vi "Configure QuickDrop UI.vi"(6 "Type":T2=enum."Double Float", 7 "FP UI References":T1, 8 "error in (no error)":errorcluster, 10 "Operation":string) -> (0 "error out":errorcluster)   [LabVIEW 2016]
doc: "Dynamically shows or hides the relevant controls on the front panel of the Quick Drop UI, and renames some of the captions for controls to make it perform correctly."
uses:
  <vilib>/Utility/Data Type/Type Definitions/Data Type.ctl
  FP UI References.ctl
  Comparison Ctrl Refs.ctl
  Comparison Captions.ctl
  Comparison Visibility.ctl
  <vilib>/Utility/Data Type/NI_Data Type.lvlib
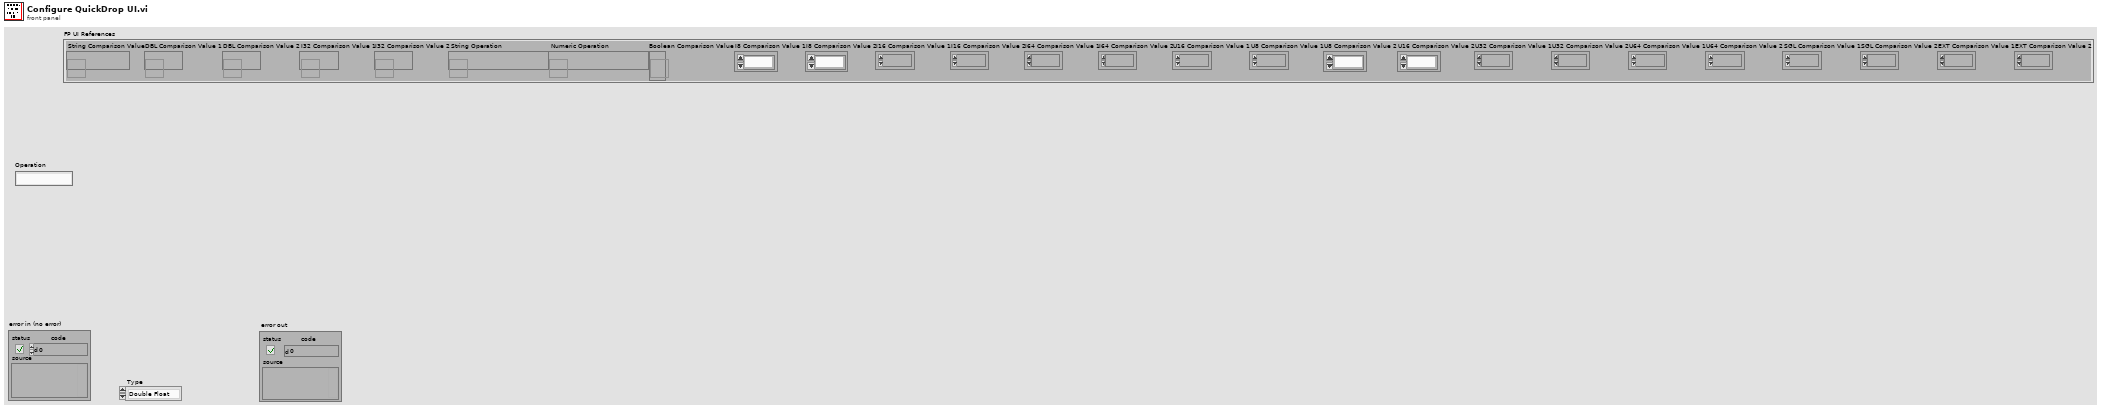
[diagram p1: front panel]
types:
  T1 = typedef "FP UI References.ctl" = cluster{"String Comparison Value":refnum<vi>, "DBL Comparison Value 1":refnum<vi>, "DBL Comparison Value 2":refnum<vi>, "I32 Comparison Value 1":refnum<vi>, "I32 Comparison Value 2":refnum<vi>, "String Operation":refnum<vi>, "Numeric Operation":refnum<vi>, "Boolean Comparison Value":refnum<vi>, "I8 Comparison Value 1":refnum<vi>, "I8 Comparison Value 2":refnum<vi>, "I16 Comparison Value 1":refnum<vi>, "I16 Comparison Value 2":refnum<vi>, "I64 Comparison Value 1":refnum<vi>, "I64 Comparison Value 2":refnum<vi>, "U16 Comparison Value 1":refnum<vi>, "U8 Comparison Value 1":refnum<vi>, "U8 Comparison Value 2":refnum<vi>, "U16 Comparison Value 2":refnum<vi>, "U32 Comparison Value 1":refnum<vi>, "U32 Comparison Value 2":refnum<vi>, "U64 Comparison Value 1":refnum<vi>, "U64 Comparison Value 2":refnum<vi>, "SGL Comparison Value 1":refnum<vi>, "SGL Comparison Value 2":refnum<vi>, "EXT Comparison Value 1":refnum<vi>, "EXT Comparison Value 2":refnum<vi>}
  T2 = typedef "NI_Data Type.lvlib/Data Type.ctl" = enum8{"Invalid Type", "Void", "I8", "I16", "I32", "I64", "U8", "U16", "U32", "U64", "Single Float", "Double Float", "Extended Float", "Single Complex", "Double Complex", "Extended Complex", "Enum U8", "Enum U16", "Enum U32", "Enum U64", "Single Float With Unit", "Double Float With Unit", "Extended Float With Unit", "Single Complex with Unit", "Double Complex with Unit", "Extended Complex with Unit", "Boolean", "String", "Path", "Picture", "Tag", "Array", "Cluster", "Variant", "LV Variant", "Waveform", "Timestamp", "Digital Waveform", "Digital Data", "ExpressData", "Refnum", "External Data", "VI", "Poly VI", "LabVIEW Class Instance", "Fixed Point"}
  T3 = typedef "Comparison Visibility.ctl" = cluster{"Comparison 2 Visible":bool, "Comparison 1 Visible":bool}
  T4 = typedef "Comparison Captions.ctl" = cluster{"Comparison 1 Caption":string, "Comparison 2 Caption":string}
  T5 = typedef "Comparison Ctrl Refs.ctl" = cluster{"Comparison Value 1 Control":refnum<vi>, "Comparison Value 2 Control":refnum<vi>}
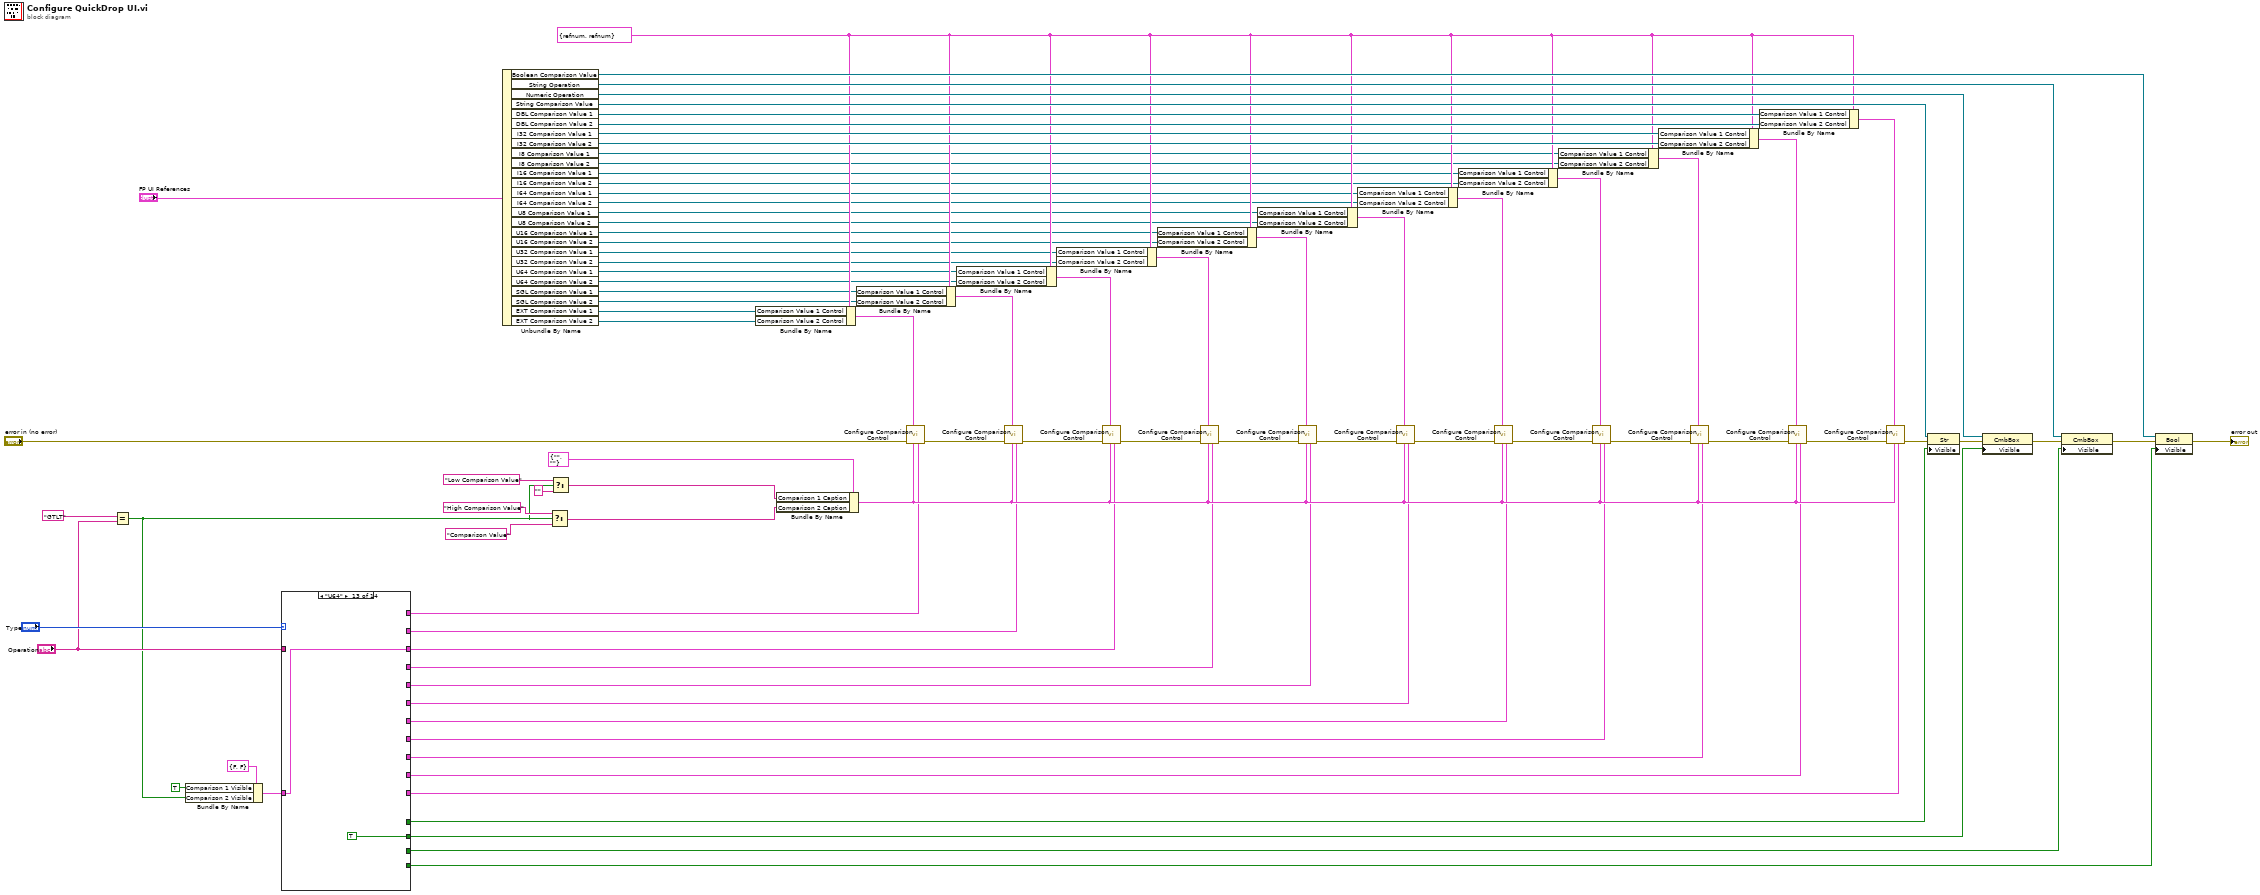
[diagram p0: block diagram]
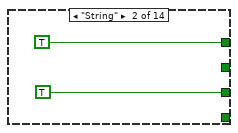
[diagram p3: hidden frame]
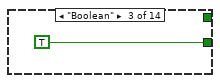
[diagram p4: hidden frame]
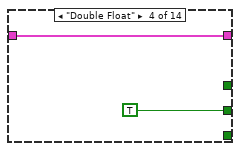
[diagram p5: hidden frame]
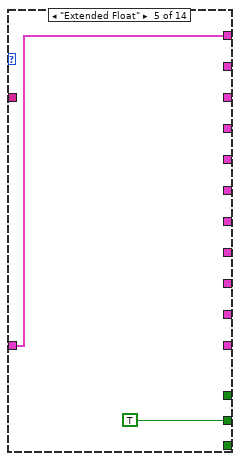
[diagram p6: hidden frame]
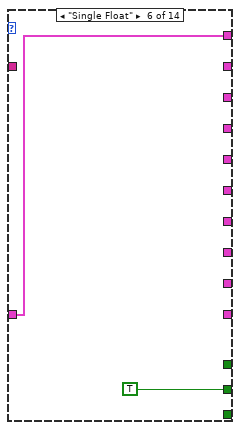
[diagram p7: hidden frame]
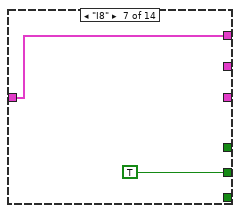
[diagram p8: hidden frame]
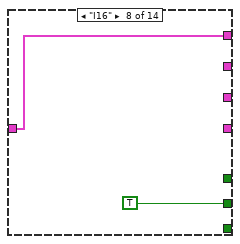
[diagram p9: hidden frame]
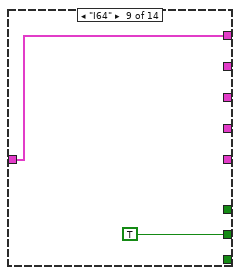
[diagram p10: hidden frame]
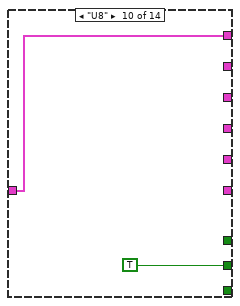
[diagram p11: hidden frame]
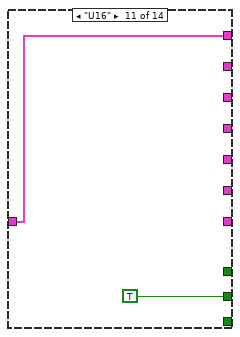
[diagram p12: hidden frame]
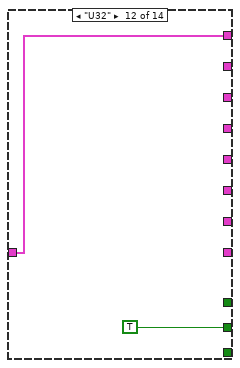
[diagram p13: hidden frame]
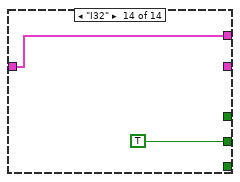
[diagram p14: hidden frame]
diagram:
  w55 = T5 {"Comparison Value 1 Control"=refnum, "Comparison Value 2 Control"=refnum} ("Control Refs")
  n1 = Equal?(x="GTLT", y="Operation") -> (x = y?=w2:bool)
  n2 = Bundle By Name(cluster=T3 {"Comparison 2 Visible"=FALSE, "Comparison 1 Visible"=FALSE} ("Control Visibility"), "Comparison 1 Visible"=TRUE, "Comparison 2 Visible"=w2) -> (w1:T3)
  n3 = case shown="\"U64\"" "Type" {
    tunnel: [_ TRUE _ _ _ _ _ _ _ _ _ _ _ _] -> w79
    tunnel: [_ TRUE _ _ _ _ _ _ _ _ _ _ _ _] -> w75
    tunnel: [_ _ _ TRUE TRUE TRUE TRUE TRUE TRUE TRUE TRUE TRUE TRUE TRUE] -> w74
    tunnel: "Operation" -> [_ _ _ _ _ _ _ _ _ _ _ _ _ _]
    tunnel: [_ _ TRUE _ _ _ _ _ _ _ _ _ _ _] -> w66
    tunnel: [_ _ _ _ w91 _ _ _ _ _ _ _ _ _] -> w15
    tunnel: [_ _ _ _ _ w93 _ _ _ _ _ _ _ _] -> w14
    tunnel: [_ _ _ _ _ _ _ _ _ _ _ _ w107 _] -> w13
    tunnel: [_ _ _ _ _ _ _ _ _ _ _ w105 _ _] -> w12
    tunnel: [_ _ _ _ _ _ _ _ _ _ w103 _ _ _] -> w11
    tunnel: [_ _ _ _ _ _ _ _ _ w101 _ _ _ _] -> w10
    tunnel: [_ _ _ _ _ _ _ _ w99 _ _ _ _ _] -> w9
    tunnel: [_ _ _ _ _ _ _ w97 _ _ _ _ _ _] -> w8
    tunnel: [_ _ _ _ _ _ w95 _ _ _ _ _ _ _] -> w7
    tunnel: [_ _ _ _ _ _ _ _ _ _ _ _ _ w109] -> w6
    tunnel: [_ _ _ w89 _ _ _ _ _ _ _ _ _ _] -> w5
    tunnel: w1 -> [_ _ _ w89 w91 w93 w95 w97 w99 w101 w103 w105 w107 w109]
    frame "Invalid Type", Default {
    }
    frame "String" {
    }
    frame "Boolean" {
    }
    frame "Double Float" {
    }
    frame "Extended Float" {
    }
    frame "Single Float" {
    }
    frame "I8" {
    }
    frame "I16" {
    }
    frame "I64" {
    }
    frame "U8" {
    }
    frame "U16" {
    }
    frame "U32" {
    }
    frame "U64" {
    }
    frame "I32" {
    }
  }
  n4 = Unbundle By Name("FP UI References") -> ("Boolean Comparison Value"=w67:refnum<vi>, "String Operation"=w76:refnum<vi>, "Numeric Operation"=w69:refnum<vi>, "String Comparison Value"=w83:refnum<vi>, "DBL Comparison Value 1"=w57:refnum<vi>, "DBL Comparison Value 2"=w56:refnum<vi>, "I32 Comparison Value 1"=w63:refnum<vi>, "I32 Comparison Value 2"=w62:refnum<vi>, "I8 Comparison Value 1"=w54:refnum<vi>, "I8 Comparison Value 2"=w53:refnum<vi>, "I16 Comparison Value 1"=w52:refnum<vi>, "I16 Comparison Value 2"=w51:refnum<vi>, "I64 Comparison Value 1"=w50:refnum<vi>, "I64 Comparison Value 2"=w49:refnum<vi>, "U8 Comparison Value 1"=w48:refnum<vi>, "U8 Comparison Value 2"=w47:refnum<vi>, "U16 Comparison Value 1"=w46:refnum<vi>, "U16 Comparison Value 2"=w45:refnum<vi>, "U32 Comparison Value 1"=w44:refnum<vi>, "U32 Comparison Value 2"=w43:refnum<vi>, "U64 Comparison Value 1"=w42:refnum<vi>, "U64 Comparison Value 2"=w41:refnum<vi>, "SGL Comparison Value 1"=w40:refnum<vi>, "SGL Comparison Value 2"=w39:refnum<vi>, "EXT Comparison Value 1"=w38:refnum<vi>, "EXT Comparison Value 2"=w37:refnum<vi>)
  n5 = Select(t="High Comparison Value", s=w2, f="Comparison Value") -> (s? t:f=w58:string)
  n6 = Select(t="Low Comparison Value", s=w2, f="") -> (s? t:f=w59:string)
  n7 = Bundle By Name(cluster=w55, "Comparison Value 1 Control"=w38, "Comparison Value 2 Control"=w37) -> (w17:T5)
  n8 = Bundle By Name(cluster=T4 {"Comparison 1 Caption"="", "Comparison 2 Caption"=""} ("Control Captions"), "Comparison 1 Caption"=w59, "Comparison 2 Caption"=w58) -> (w16:T4)
  n9 = Bundle By Name(cluster=w55, "Comparison Value 1 Control"=w40, "Comparison Value 2 Control"=w39) -> (w19:T5)
  n10 = call "Configure Comparison Control.vi"("Control Visibility"=w15, "Control Captions"=w16, "Control Refs"=w17, "error in (no error)"="error in (no error)") -> ("error out"=w18:errorcluster)  [unwired: 7 in]
  n11 = Bundle By Name(cluster=w55, "Comparison Value 1 Control"=w42, "Comparison Value 2 Control"=w41) -> (w20:T5)
  n12 = call "Configure Comparison Control.vi"("Control Visibility"=w14, "Control Captions"=w16, "Control Refs"=w19, "error in (no error)"=w18) -> ("error out"=w35:errorcluster)  [unwired: 7 in]
  n13 = Bundle By Name(cluster=w55, "Comparison Value 1 Control"=w44, "Comparison Value 2 Control"=w43) -> (w21:T5)
  n14 = call "Configure Comparison Control.vi"("Control Visibility"=w13, "Control Captions"=w16, "Control Refs"=w20, "error in (no error)"=w35) -> ("error out"=w28:errorcluster)  [unwired: 7 in]
  n15 = Bundle By Name(cluster=w55, "Comparison Value 1 Control"=w46, "Comparison Value 2 Control"=w45) -> (w22:T5)
  n16 = call "Configure Comparison Control.vi"("Control Visibility"=w12, "Control Captions"=w16, "Control Refs"=w21, "error in (no error)"=w28) -> ("error out"=w30:errorcluster)  [unwired: 7 in]
  n17 = Bundle By Name(cluster=w55, "Comparison Value 1 Control"=w48, "Comparison Value 2 Control"=w47) -> (w23:T5)
  n18 = call "Configure Comparison Control.vi"("Control Visibility"=w11, "Control Captions"=w16, "Control Refs"=w22, "error in (no error)"=w30) -> ("error out"=w29:errorcluster)  [unwired: 7 in]
  n19 = Bundle By Name(cluster=w55, "Comparison Value 1 Control"=w50, "Comparison Value 2 Control"=w49) -> (w24:T5)
  n20 = call "Configure Comparison Control.vi"("Control Visibility"=w10, "Control Captions"=w16, "Control Refs"=w23, "error in (no error)"=w29) -> ("error out"=w34:errorcluster)  [unwired: 7 in]
  n21 = Bundle By Name(cluster=w55, "Comparison Value 1 Control"=w52, "Comparison Value 2 Control"=w51) -> (w25:T5)
  n22 = call "Configure Comparison Control.vi"("Control Visibility"=w9, "Control Captions"=w16, "Control Refs"=w24, "error in (no error)"=w34) -> ("error out"=w31:errorcluster)  [unwired: 7 in]
  n23 = Bundle By Name(cluster=w55, "Comparison Value 1 Control"=w54, "Comparison Value 2 Control"=w53) -> (w26:T5)
  n24 = call "Configure Comparison Control.vi"("Control Visibility"=w8, "Control Captions"=w16, "Control Refs"=w25, "error in (no error)"=w31) -> ("error out"=w33:errorcluster)  [unwired: 7 in]
  n25 = Bundle By Name(cluster=w55, "Comparison Value 1 Control"=w63, "Comparison Value 2 Control"=w62) -> (w61:T5)
  n26 = call "Configure Comparison Control.vi"("Control Visibility"=w7, "Control Captions"=w16, "Control Refs"=w26, "error in (no error)"=w33) -> ("error out"=w32:errorcluster)  [unwired: 7 in]
  n27 = Bundle By Name(cluster=w55, "Comparison Value 1 Control"=w57, "Comparison Value 2 Control"=w56) -> (w27:T5)
  n28 = call "Configure Comparison Control.vi"("Control Visibility"=w6, "Control Captions"=w16, "Control Refs"=w61, "error in (no error)"=w32) -> ("error out"=w81:errorcluster)  [unwired: 7 in]
  n29 = call "Configure Comparison Control.vi"("Control Visibility"=w5, "Control Captions"=w16, "Control Refs"=w27, "error in (no error)"=w81) -> ("error out"=w36:errorcluster)  [unwired: 7 in]
  n30 = property class="Str"(reference=w83, error in=w36, "Visible"=w79) -> (error out=w80:errorcluster)  [unwired: 1 out]
  n31 = property class="CmbBox"(reference=w69, error in=w80, "Visible"=w74) -> (error out=w78:errorcluster)  [unwired: 1 out]
  n32 = property class="CmbBox"(reference=w76, error in=w78, "Visible"=w75) -> (error out=w77:errorcluster)  [unwired: 1 out]
  n33 = property class="Bool"(reference=w67, error in=w77, "Visible"=w66) -> (error out=→"error out":errorcluster)  [unwired: 1 out]
